vi "2_Waveform_Signal_Classification(Inference).vi"() -> ()   [LabVIEW 2020]
uses:
  <vilib>/Ngene/DeepLTK/Toolkit/NN_Network/Controls/NN_Save_Before_Destroy_Options.ctl
  <vilib>/Ngene/DeepLTK/Toolkit/NN_Layers/Layers/Input/API/NN_Layer_Set_Out(Input1D_idx).vi
  <vilib>/Ngene/DeepLTK/Toolkit/Deep_Learning_Toolkit_by_Ngene.lvlib
  <vilib>/measure/NI_MABase.lvlib
panel:
  out "Predicted Class":string="Triangle Wave"
  out "Class Labels":string[](array[string])=["Triangle Wave", "Square Wave", "Sine Wave", "Sawtooth Wave", "Noise"]
  in  "Offset":dbl(slide)=-0.6870229007633579 scale=-10.0..10.0
  out "Generated WaveForm":waveform(dbl)(graph)={"t0"=timestamp(0 s since 1904-01-01), "dt"=0.001, "Y"=[-4.376143581376376, -5.740333313909443, -4.200321659576944, -2.6603100052444444, -1.1202983509119497, 0.41971330342054824, 1.9597249577530471, 3.499736612085546, 3.868648680146845, 2.3286370258143467, 0.7886253714818474, -0.7513862828506518, -2.2913979371831488, -3.8314095915156483, -5.371421245848147, -4.745055649437671, -3.2050439951051795, -1.6650323407726821, -0.1250206864401836, 1.4149909678923152, 2.955002622224814, 4.413382670007574, 2.8733710156750747, 1.3333593613425765, -0.20665229298992266, -1.7466639473224208, -3.28667560165492, -4.826687255987419, -5.289789639298402, -3.7497779849659025, -2.2097663306334034, -0.6697546763009188, 0.870256978031593, 2.4102686323640783, 3.9502802866965903, 3.4181050055358106, 1.8780933512032987, 0.33808169687081335, -1.201929957461686, -2.7419416117941853, -4.281953266126682, -5.821964920459181, -4.294511974826637, -2.754500320494138, -1.2144886661616412, 0.3255229881708577, 1.8655346425033565, 3.4055462968358547, 3.962838995396533, 2.4228273410640337, 0.8828156867315355, -0.6571959676009638, -2.1972076219334618, -3.7372192762659613, -5.277230930598461, -4.839245964687361, -3.2992343103548616, -1.7592226560223623, -0.21921100168986446, 1.3208006526426344, 2.8608123069751334, 4.400823961307619, 2.9675613309247697, 1.4275496765922706, -0.11246197774022781, -1.6524736320727271, -3.192485286405226, -4.732496940737712, -5.383979954548096, -3.843968300215583, -2.303956645883097, -0.7639449915506116, 0.7760666627818991, 2.316078317114411, 3.856089971446896, 3.5122953207855048, 1.9722836664529928, 0.43227201212048083, -1.1077396422119785, -2.6477512965444916, -4.187762950877002, -5.727774605209513, -4.3887022900763455, -2.848690635743832, -1.3086789814113213, 0.23133267292118986, 1.7713443272536495, 3.311355981586161, 4.057029310646213, 2.5170176563137026, 0.9770060019812419, -0.56300565235127, -2.103017306683782, -3.6430289610162925, -5.183040615348753, -4.933436279937054, -3.3934246256045415, -1.853412971272031, -0.31340131693957135, 1.2266103373929405]}
  in  "Phase":dbl(slide)=244.58015267175574 scale=0.0..360.0
  in  "Signal Type":T1(ring)=enum."Triangle Wave"
  in  "Amplitude":dbl(slide)=5.141221374045801 scale=0.2..10.0
  in  "Frequency":dbl(slide)=74.88549618320612 scale=10.0..100.0
  in  "Weight File Path":path=path "D:/Ngene/GitHub/deepltk_examples/2_Waveform_Processing/21_Waveform_Signal_Classifier/working/WF_Classifier/WF_Classifier_weights_23_10_04__16_17_04.bin"
  in  "Configuration File Path":path=path "D:/Ngene/GitHub/deepltk_examples/2_Waveform_Processing/21_Waveform_Signal_Classifier/working/WF_Classifier/WF_Classifier_net_cfg_23_10_04__16_17_04.cfg"
  out "Class Probabilities":sgl[](array[slide])=[1.0, 7.697561e-18, 5.7099507e-15, 0.0, 0.0] scale=0.0..1.0
  in  "Stop":bool
  # "Overview: Demonstrates the usage of DeepLTK for loading the model pretrained for waveform signal classification and running for inference.\nRequirements: DeepLTK - Deep Learning Toolkit for LabVIEW (https://www.ngene.co/deep-learning-toolkit-for-labview)\nInstructions:\n1. Provide Network Configuration File Path and Weight File Path generated from training example.\n2. Run the VI\n3. Input Waveform parameters and observe the predicted frequency against reference value.\n4. Press the Stop button to stop the VI.\n\nMore Examples:  https://github.com/ngenehub/deepltk_examples"
  # "1D Waveform Signal Clasification Inference Demo"
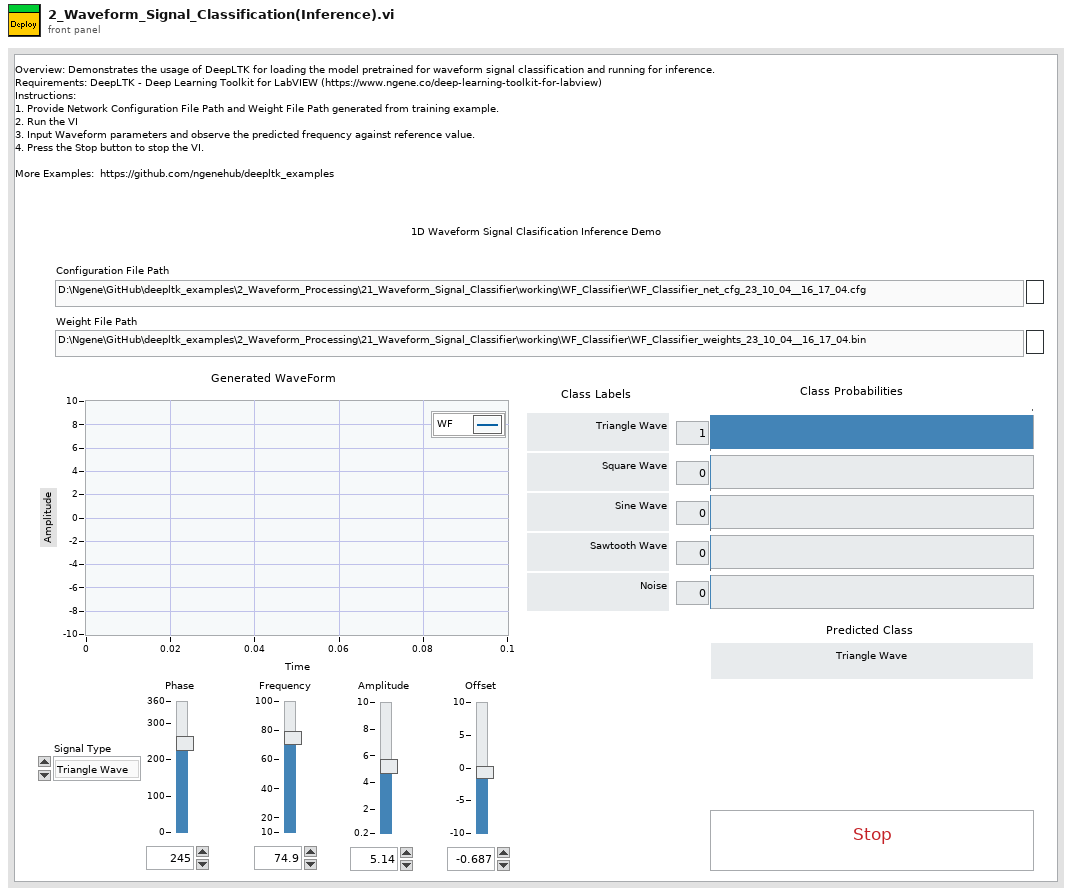
[diagram p1: front panel]
types:
  T1 = enum16{"Sine Wave", "Triangle Wave", "Square Wave", "Sawtooth Wave", "Noise"}
  T2 = typedef "Deep_Learning_Toolkit_by_Ngene.lvlib/NN_Save_Before_Destroy_Options.ctl" = cluster{"CFG?":bool, "Weights?":bool, "Render?":bool}
  T3 = typedef "Deep_Learning_Toolkit_by_Ngene.lvlib/NN_Config_Params.ctl" = cluster{"Name":string, "mBatch":i32, "NN_Train_Params":T4, "LR_Decay_Policy":T7, "Labels":string[], "Loss":T9}
  T4 = typedef "Deep_Learning_Toolkit_by_Ngene.lvlib/NN_Train_Params.ctl" = cluster{"Optimizer":T5, "Beta_1":sgl, "Beta_2":sgl, "Weight Decay(L1)":sgl, "Weight Decay(L2)":sgl, "Data_Sampling":T6}
  T5 = typedef "Deep_Learning_Toolkit_by_Ngene.lvlib/NN_Train_Optimizer.ctl" = enum16{"SGD", "Adam", "Adagrad", "Adadelta", "RMSProp", "Nesterov"}
  T6 = typedef "Deep_Learning_Toolkit_by_Ngene.lvlib/NN_Train_Data_Sampling.ctl" = enum16{"Random", "Sequential"}
  T7 = typedef "Deep_Learning_Toolkit_by_Ngene.lvlib/NN_LR_Policy_Cfg.ctl" = cluster{"Policy_Type":T8, "LR0":dbl, "k":sgl, "WarmUp_Policy":enum16{"Step", "Ramp"}, "WarmUp_Iter":i32, "WarmUp_Ratio":sgl}
  T8 = typedef "Deep_Learning_Toolkit_by_Ngene.lvlib/NN_LR_Policy_Type.ctl" = enum16{"Manual", "Step", "Exp", "1/t"}
  T9 = typedef "Deep_Learning_Toolkit_by_Ngene.lvlib/NN_Loss_Config_Params.ctl" = cluster{"Loss_Type":T10, "Loss_Conf_Params":variant}
  T10 = typedef "Deep_Learning_Toolkit_by_Ngene.lvlib/NN_Loss_Type.ctl" = enum16{"None", "MSE", "CrossEntropy", "YOLO_v2"}
  T11 = typedef "Deep_Learning_Toolkit_by_Ngene.lvlib/NN_Layer_Config_Params.ctl" = cluster{"Layer_Type":T12, "Layer_Conf_Params":variant}
  T12 = typedef "Deep_Learning_Toolkit_by_Ngene.lvlib/NN_Layer_Type.ctl" = enum16{"Input1D", "Input3D", "Conv2D", "Conv2D_Adv", "MaxPool", "AvgPool", "UpSample", "DropOut3D", "ShortCut", "Concat", "SoftMax3D", "FC", "DropOut", "Softmax", "Flatten", "YOLO_v2", "Unsupported"}
  T13 = typedef "Deep_Learning_Toolkit_by_Ngene.lvlib/NN.ctl" = cluster{"Name":string, "No of Layers":i32, "mBatch":i32, "Layers":T14[], "Dimty":T15, "Dims_In":T16, "Dims_Out":T16, "Working_Dir":path, "Train?":bool, "Train_Params":T4, "LR_Update_Policy":T7, "Session Data":T17, "Ground_truth":T18, "NNg_hdls":T20, "NN_Device":T21, "GPU Id":i32, "Labels":string[], "Receptive Field":T22[], "Loss_Type":T10, "Loss_Cfg_Prms":variant}
  T14 = typedef "Deep_Learning_Toolkit_by_Ngene.lvlib/NN_Layer_ref.ctl" = refnum<data-value>
  T15 = typedef "Deep_Learning_Toolkit_by_Ngene.lvlib/NN_In_Out_Dim-ty.ctl" = enum8{"In1D_Out1D", "In3D_Out1D", "In3D_Out3D", "In3D_OutBBox"}
  T16 = typedef "Deep_Learning_Toolkit_by_Ngene.lvlib/NN_Dims(C,H,W).ctl" = cluster{"C":i32, "H":i32, "W":i32}
  T17 = typedef "Deep_Learning_Toolkit_by_Ngene.lvlib/NN_Train_Session_Data.ctl" = cluster{"Epochs":sgl, "Tot_Iter":i32, "LR":sgl, "LR_iter":i32}
  T18 = typedef "Deep_Learning_Toolkit_by_Ngene.lvlib/NN_Ground_truth.ctl" = cluster{"Y":variant, "Y_idx":T19}
  T19 = typedef "Deep_Learning_Toolkit_by_Ngene.lvlib/NN_Data_ref(1D_I32).ctl" = refnum<data-value>
  T20 = typedef "Deep_Learning_Toolkit_by_Ngene.lvlib/nng_cuda_handles.ctl" = cluster{"cudnn":u64, "cublas":u64, "stream":u64, "curand":u64}
  T21 = typedef "Deep_Learning_Toolkit_by_Ngene.lvlib/NN_Device.ctl" = enum16{"CPU", "GPU"}
  T22 = typedef "Deep_Learning_Toolkit_by_Ngene.lvlib/NN_Dims(V,H).ctl" = cluster{"V":i32, "H":i32}
  T23 = typedef "Deep_Learning_Toolkit_by_Ngene.lvlib/NN_Layer.ctl" = cluster{"Name":string, "Layer_Data":variant, "Layer_Type":T12, "Dims_In":T16, "Layers_In":variant, "Dims_Out":T16, "Layers_Out":variant, "Metrics":T24, "GPU_Data":variant, "mBatch":i32, "NN_Device":T21, "NNg_hdls":T20, "Train?":bool, "Dimty":T25, "RecptField":T26}
  T24 = typedef "Deep_Learning_Toolkit_by_Ngene.lvlib/NN_Layer_Metrics.ctl" = cluster{"Data":dbl, "Params":dbl, "Ops":dbl}
  T25 = typedef "Deep_Learning_Toolkit_by_Ngene.lvlib/NN_Layer_Dimty.ctl" = enum16{"1D", "3D"}
  T26 = typedef "Deep_Learning_Toolkit_by_Ngene.lvlib/NN_Layer_RF_State.ctl" = cluster{"Dims":T22, "J":T22}
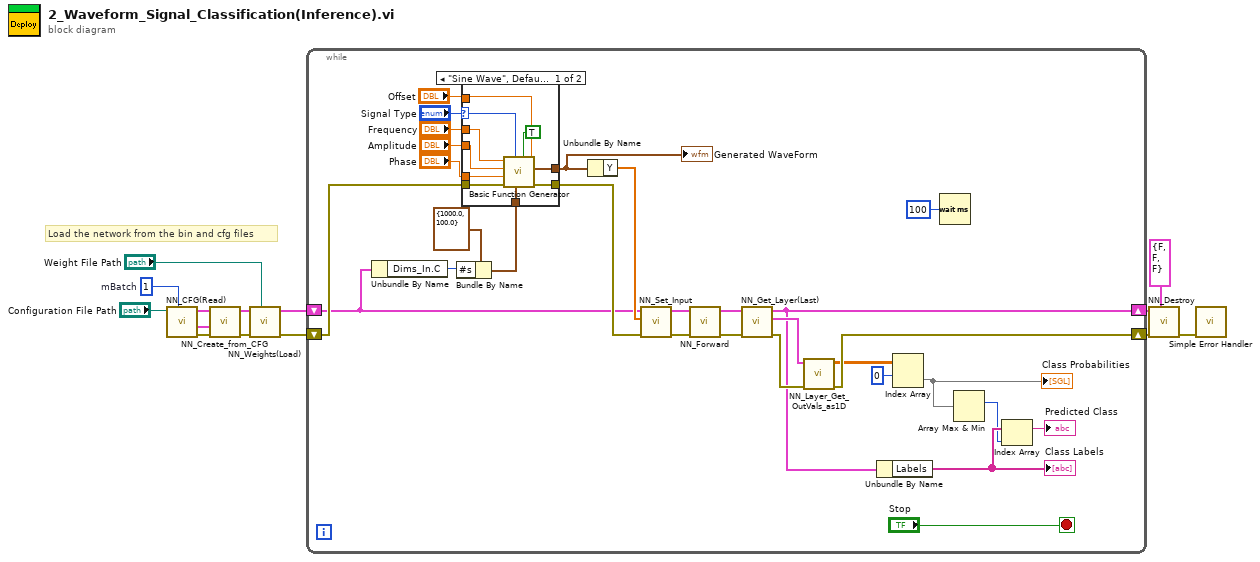
[diagram p0: block diagram]
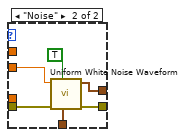
[diagram p2: hidden frame]
diagram:
  w1 = 1  # mBatch
  # "Load the network from the bin and cfg files"
  n1 = call <vilib>:"NN_CFG(Read).vi"("mBatch"=w1, "CFG file path"="Configuration File Path") -> ("error out"=w8:errorcluster, "Net_Cfg"=w9:T3, "Layer_Cfg"=w7:T11[])  [unwired: 7 in]
  n2 = call <vilib>:"NN_Create_from_CFG.vi"("error in (no error)"=w8, "Net_Cfg"=w9, "Layer_Cfg"=w7) -> ("error out"=w11:errorcluster, "NN out"=w6:T13)  [unwired: 7 in]
  n3 = call <vilib>:"NN_Weights(Load).vi"("Weight File Path"="Weight File Path", "error in (no error)"=w11, "NN in"=w6) -> ("error out"=w5:errorcluster, "NN out"=w4:T13)  [unwired: 7 in]
  n4 = while {
    shift-right: [w42] -> w14
    shift-left: w5 -> [w43]
    shift-right: [w21] -> w13
    shift-left: w4 -> [w24]
    stop <- "Stop" stop-if-true
    n5 = Unbundle By Name(w24) -> ("Dims_In.C"=w22:i32)
    n6 = Bundle By Name(cluster=cluster{"Fs":dbl, "#s":dbl} {"Fs"=1000.0, "#s"=100.0} ("sampling info"), "#s"=w22) -> (w23:cluster{"Fs":dbl, "#s":dbl})
    n7 = case shown="\"Sine Wave\", Default" "Signal Type" {
      selector: "Signal Type" -> [w48 _]
      tunnel: w43 -> [w53 w59]
      tunnel: "Frequency" -> [w52 _]
      tunnel: "Amplitude" -> [w51 w54]
      tunnel: [w50 w56] -> w31
      tunnel: [w49 w57] -> w19
      tunnel: "Phase" -> [w47 _]
      tunnel: "Offset" -> [w46 _]
      tunnel: w23 -> [w44 w58]
      frame "Sine Wave", Default {
        n8 = call <vilib>:"Basic Function Generator.vi"("offset"=w46, "reset signal"=TRUE, "sampling info"=w44, "signal type"=w48, "error in (no error)"=w53, "phase"=w47, "amplitude"=w51, "frequency"=w52) -> ("error out"=w50:errorcluster, "signal out"=w49:waveform(dbl))  [unwired: 1 in, 1 out]
      }
      frame "Noise" {
        n9 = call <vilib>:"Uniform White Noise Waveform.vi"("sampling info"=w58, "reset signal"=TRUE, "error in (no error)"=w59, "amplitude"=w54) -> ("error out"=w56:errorcluster, "signal out"=w57:waveform(dbl))  [unwired: 6 in]
      }
    }
    "Generated WaveForm" <- w19
    n10 = Unbundle By Name(w19) -> ("Y"=w30:dbl[])
    n11 = call-poly <vilib>:"NN_Set_Input.vi"("error in (no error)"=w31, "Data_In(1D_SGL)"=w30, "NN In"=w24) -> ("error out"=w41:errorcluster, "NN Out"=w38:T13)  [unwired: 7 in]
    n12 = call <vilib>:"NN_Forward.vi"("error in (no error)"=w41, "NN in"=w38) -> ("error out"=w40:errorcluster, "NN out"=w39:T13)  [unwired: 6 in, 2 out]
    n13 = call <vilib>:"NN_Get_Layer(Last).vi"("error in (no error)"=w40, "NN in"=w39) -> ("error out"=w37:errorcluster, "Last_Layer"=w36:T23, "NN out"=w21:T13)  [unwired: 6 in, 1 out]
    n14 = call <vilib>:"NN_Layer_Get_OutVals_as1D.vi"("error in (no error)"=w37, "Layer"=w36) -> ("error out"=w42:errorcluster, "Out(as1D)"=w35:sgl[][])  [unwired: 8 in]
    n15 = Unbundle By Name(w21) -> ("Labels"=w17:string[])
    "Class Labels" <- w17
    n16 = Index Array(array=w35, index (row)=0) -> (element=w18:sgl[])  [unwired: 1 in]
    "Class Probabilities" <- w18
    n17 = Wait (ms)(milliseconds to wait=u32 100) -> ()  [unwired: 1 out]
    n18 = Array Max & Min(array=w18) -> (max index (indices)=w16:i32)  [unwired: 3 out]
    n19 = Index Array(array=w17, index=w16) -> (element=→"Predicted Class":string)
  }
  n20 = call <vilib>:"NN_Destroy.vi"("Save (T, T, T)"=T2 {"CFG?"=FALSE, "Weights?"=FALSE, "Render?"=FALSE}, "error in (no error)"=w14, "NN in"=w13) -> ("error out"=w2:errorcluster)  [unwired: 8 in]
  n21 = call <vilib>:"Simple Error Handler.vi"("error in (no error)"=w2) -> ()  [unwired: 4 in, 5 out]
